vi "Read U64 Direct.vi"(8 "error in (no error)":errorcluster, 9 "Timeout (ms)":i32, 11 "CIFTag in":refnum<class "CIF_CIPC_Chn_U64.lvclass">) -> (0 "error out":errorcluster, 1 "timed out?":bool, 2 "Data":u64, 3 "CIFTag out":refnum<class "CIF_CIPC_Chn_U64.lvclass">)   [LabVIEW 2021, in "CIF_CIPC_Chn_U64.lvclass"]
uses:
  CIF_CIPC_Chn_U64.lvclass
  D:/dev/Packages/CIF_Channels_Core/src/CIFChannels/CIFChannels.lvclass
  D:/dev/Packages/CIF_Channels_Core/src/CIPC_Channels/CIF_CIPC_Chan/CIF_CIPC_Chn.lvclass
  CIFChannels/CIFChannels.lvclass/CIFChannels.ctl
  CIFChannels/Typedef/Channel State.ctl
  CIFChannels/Typedef/Direction.ctl
  CIF_CIPC_Chn_U64.lvclass/CIF_CIPC_Chn_U64.ctl
  CIF_CIPC_Chan/CIF_CIPC_Chn.lvclass/CIF_CIPC_Chn.ctl
  <vilib>/CIF Foundation/CIF CIPC/TypeDefs/Data Element Details.ctl
  ed3b2614-2534-48bf-9d55-8103b1731be4.vi
  9835d51f-0a03-4fca-8b65-57ff329e3dc0.vi
  09931085-5d07-4563-aebb-184aa810b238.vi
  a8b9b8b0-6f0e-468c-aa0e-dfff2efe2781.vi
  CIF_CIPC_Chan/Accessors/Read Buffer Configuration.vi
  CIF_CIPC_Chan/Accessors/Read Data Type.vi
  CIFChannels/Accessors/Read Channel State.vi
  CIFChannels/Accessors/Read Direction.vi
  CIFChannels/Accessors/Read Tag Forced.vi
  CIFChannels/Accessors/Write Channel State.vi
  CIFChannels/Accessors/Read Tag Disconnect Behavior.vi
  <vilib>/CIF Foundation/CIF CIPC/SubVIs/Wait For N Elements Available.vi
  <vilib>/CIF Foundation/CIF CIPC/SubVIs/Get Element Read Position.vi
  <vilib>/CIF Foundation/CIF CIPC/SubVIs/Check Error.vi
  <vilib>/CIF Foundation/CIF CIPC/SubVIs/Get dll Path.vi
  <vilib>/CIF Foundation/CIF CIPC/SubVIs/Set Element Read Position.vi
  CIF_CIPC_Chan/CIF_CIPC_Chn.lvclass
  <vilib>/Utility/error.llb/Trim Whitespace.vi
  <vilib>/Utility/error.llb/Error Cluster From Error Code.vi
  CIFChannels/CIFChannels.lvclass
  <vilib>/CIF Foundation/CIF CIPC/CIF_NI_CIPC.lvlib
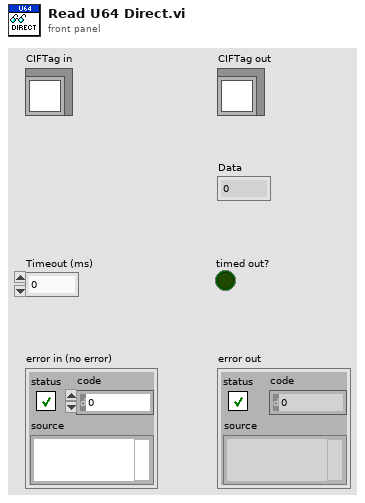
[diagram p1: front panel]
types:
  T1 = typedef "CIFChannels.lvclass/Channel State.ctl" = enum16{"Creating", "Disconnected", "Connecting", "Connected", "Destroyed"}
  T2 = typedef "CIFChannels.lvclass/Direction.ctl" = enum16{"Publisher", "Subscriber"}
  T3 = typedef "CIF_NI_CIPC.lvlib/Data Element Details.ctl" = cluster{"Bytes to Read":u32, "Element Offset":u32}
  T4 = typedef "CIF_CIPC_Chn.lvclass/Buffer Configuration Data.ctl" = cluster{"Total Size":u32, "Read Size":u32, "Read Offset":u32, "CIPC BP References":T5, "Override CIPC Name":string, "Encoder Data":string}
  T5 = typedef "CIF_NI_CIPC.lvlib/Backpressure References.ctl" = cluster{"CIPC Reference":u64, "CIPC BP Reference":u64}
  T6 = typedef "NI_Data Type.lvlib/Data Type.ctl" = enum8{"Invalid Type", "Void", "I8", "I16", "I32", "I64", "U8", "U16", "U32", "U64", "Single Float", "Double Float", "Extended Float", "Single Complex", "Double Complex", "Extended Complex", "Enum U8", "Enum U16", "Enum U32", "Enum U64", "Single Float With Unit", "Double Float With Unit", "Extended Float With Unit", "Single Complex with Unit", "Double Complex with Unit", "Extended Complex with Unit", "Boolean", "String", "Path", "Picture", "Tag", "Array", "Cluster", "Variant", "LV Variant", "Waveform", "Timestamp", "Digital Waveform", "Digital Data", "ExpressData", "Refnum", "External Data", "VI", "Poly VI", "LabVIEW Class Instance", "Fixed Point", "Set Collection", "Map Collection"}
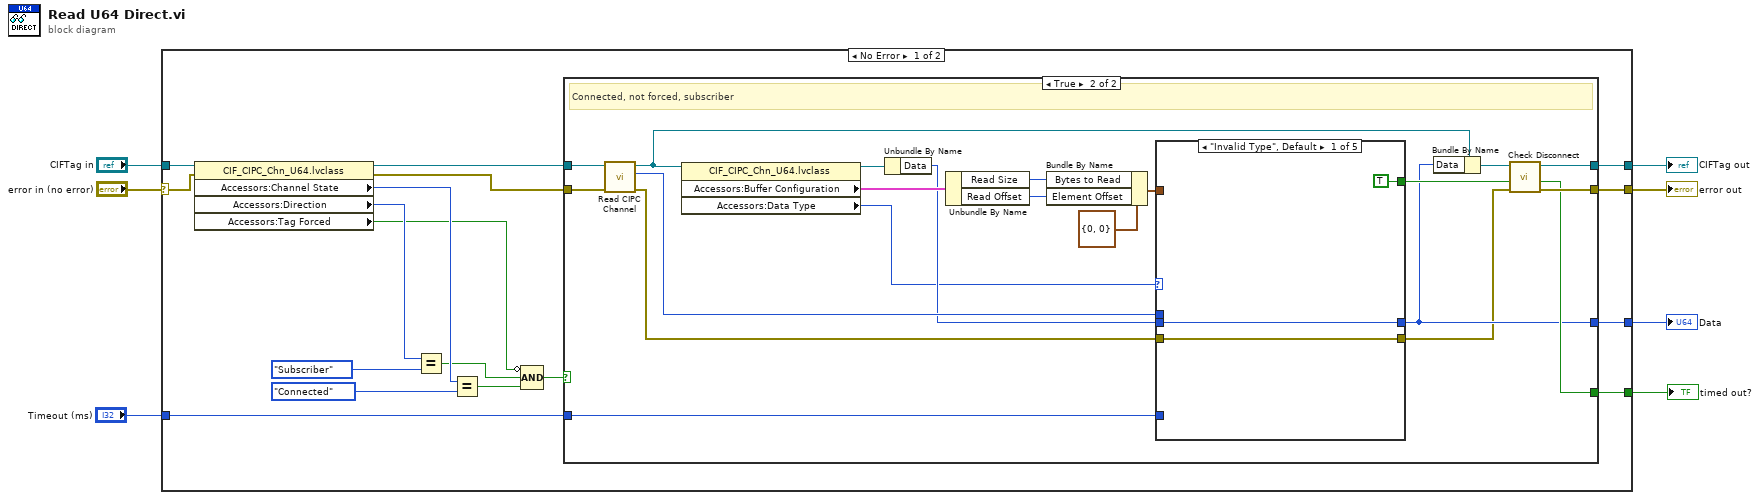
[diagram p0: block diagram]
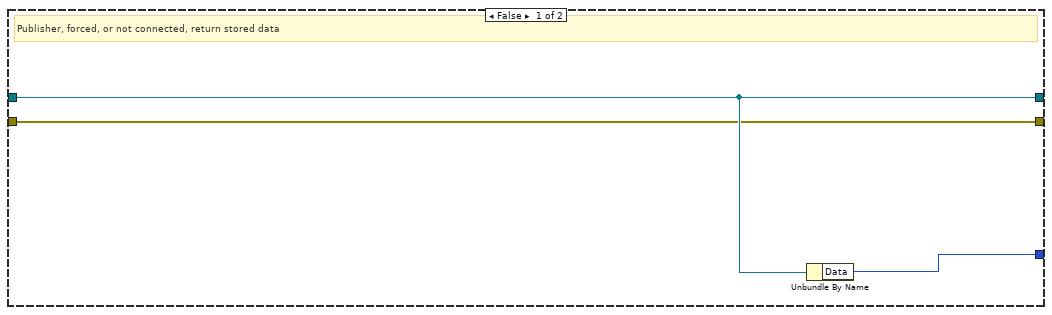
[diagram p2: hidden frame]
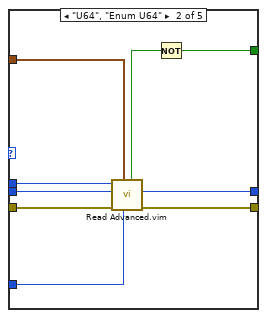
[diagram p3: hidden frame]
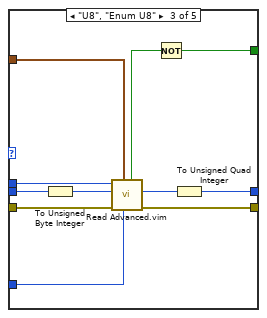
[diagram p4: hidden frame]
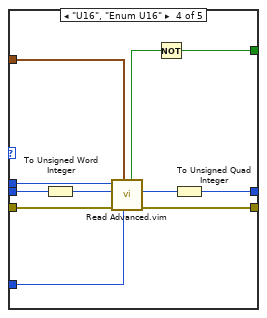
[diagram p5: hidden frame]
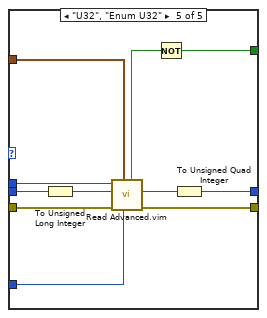
[diagram p6: hidden frame]
diagram:
  n1 = case shown="No Error" "error in (no error)" {
    selector: "error in (no error)" -> [w21 w95]
    tunnel: [w10 w95] -> w6
    tunnel: [w11 w94] -> w4
    tunnel: "CIFTag in" -> [w22 w94]
    tunnel: [w24 _] -> w3
    tunnel: [w23 _] -> w2
    tunnel: "Timeout (ms)" -> [w9 _]
    frame No Error {
      n2 = property class="CIF_CIPC_Chn_U64.lvclass"(reference=w22, error in=w21) -> (reference out=w20:refnum<class "CIF_CIPC_Chn_U64.lvclass">, error out=w19:errorcluster, "Accessors:Channel State"=w16:T1, "Accessors:Direction"=w18:T2, "Accessors:Tag Forced"=w8:bool)
      n3 = Equal?(x=w18, y=Direction."Subscriber") -> (x = y?=w12:bool)
      n4 = Equal?(x=w16, y=Channel_State."Connected") -> (x = y?=w14:bool)
      n5 = Compound Arithmetic op=AND(invert w8, w12, w14) -> (w13:bool)
      n6 = case shown="True" w13 {
        tunnel: [_ w42] -> w24
        tunnel: [w27 w31] -> w23
        tunnel: w19 -> [w25 w47]
        tunnel: w20 -> [w26 w48]
        tunnel: [w26 w45] -> w11
        tunnel: [w25 w46] -> w10
        tunnel: w9 -> [_ w32]
        frame False {
          # "Publisher, forced, or not connected, return stored data"
          n7 = Unbundle By Name(w26) -> ("Data"=w27:u64)
        }
        frame True {
          # "Connected, not forced, subscriber"
          n8 = call "Read CIPC Channel.vi"("error in (no error)"=w47, "CIFTag in"=w48) -> ("error out"=w33:errorcluster, "CIPC Channel"=w34:u64, "CIFTag out"=w41:refnum<class "CIF_CIPC_Chn_U64.lvclass">)  [unwired: 7 in]
          n9 = property class="CIF_CIPC_Chn_U64.lvclass"(reference=w41) -> (reference out=w40:refnum<class "CIF_CIPC_Chn_U64.lvclass">, "Accessors:Buffer Configuration"=w36:T4, "Accessors:Data Type"=w28:T6)  [unwired: 1 in, 1 out]
          n10 = Unbundle By Name(w40) -> ("Data"=w30:u64)
          n11 = Unbundle By Name(w36) -> ("Read Size"=w38:u32, "Read Offset"=w37:u32)
          n12 = Bundle By Name(cluster=T3 {"Bytes to Read"=0, "Element Offset"=0} ("Data Element"), "Bytes to Read"=w38, "Element Offset"=w37) -> (w35:T3)
          n13 = case shown="\"Invalid Type\", Default" w28 {
            tunnel: [TRUE w60 w71 w82 w93] -> w43
            tunnel: w35 -> [_ w59 w70 w81 w92]
            tunnel: w34 -> [_ w58 w69 w80 w91]
            tunnel: w33 -> [w50 w57 w68 w79 w90]
            tunnel: w32 -> [_ w56 w67 w78 w89]
            tunnel: [w51 w54 w61 w72 w83] -> w31
            tunnel: w30 -> [w51 w53 w64 w75 w86]
            tunnel: [w50 w52 w63 w74 w85] -> w29
            frame "Invalid Type", Default {
            }
            frame "U64", "Enum U64" {
              n14 = call "Read Advanced.vim"("Timeout (ns)"=w56, "Data Element"=w59, "error in (no error)"=w57, "Data in"=w53, "CIPC Reference in"=w58) -> ("error out"=w52:errorcluster, "Data out"=w54:u64, "Success"=w55:bool)  [unwired: 2 in, 2 out]
              n15 = Not(x=w55) -> (.not. x?=w60:bool)
            }
            frame "U8", "Enum U8" {
              n16 = To Unsigned Byte Integer(number=w64) -> (unsigned 8bit integer=w62:u8)
              n17 = call "Read Advanced.vim"("Timeout (ns)"=w67, "Data Element"=w70, "error in (no error)"=w68, "Data in"=w62, "CIPC Reference in"=w69) -> ("error out"=w63:errorcluster, "Data out"=w65:u8, "Success"=w66:bool)  [unwired: 2 in, 2 out]
              n18 = Not(x=w66) -> (.not. x?=w71:bool)
              n19 = To Unsigned Quad Integer(1:w65) -> (0:w61:u64)
            }
            frame "U16", "Enum U16" {
              n20 = To Unsigned Word Integer(number=w75) -> (unsigned 16bit integer=w73:u16)
              n21 = call "Read Advanced.vim"("Timeout (ns)"=w78, "Data Element"=w81, "error in (no error)"=w79, "Data in"=w73, "CIPC Reference in"=w80) -> ("error out"=w74:errorcluster, "Data out"=w76:u16, "Success"=w77:bool)  [unwired: 2 in, 2 out]
              n22 = Not(x=w77) -> (.not. x?=w82:bool)
              n23 = To Unsigned Quad Integer(1:w76) -> (0:w72:u64)
            }
            frame "U32", "Enum U32" {
              n24 = To Unsigned Long Integer(number=w86) -> (unsigned 32bit integer=w84:u32)
              n25 = call "Read Advanced.vim"("Timeout (ns)"=w89, "Data Element"=w92, "error in (no error)"=w90, "Data in"=w84, "CIPC Reference in"=w91) -> ("error out"=w85:errorcluster, "Data out"=w87:u32, "Success"=w88:bool)  [unwired: 2 in, 2 out]
              n26 = Not(x=w88) -> (.not. x?=w93:bool)
              n27 = To Unsigned Quad Integer(1:w87) -> (0:w83:u64)
            }
          }
          n28 = Bundle By Name(cluster=w41, "Data"=w31) -> (w44:refnum<class "CIF_CIPC_Chn_U64.lvclass">)
          n29 = call "Check Disconnect.vi"("error in (no error)"=w29, "timeout in"=w43, "CIFTag in"=w44) -> ("error out"=w46:errorcluster, "timeout out"=w42:bool, "CIFTag out"=w45:refnum<class "CIF_CIPC_Chn_U64.lvclass">)  [unwired: 5 in, 1 out]
        }
      }
    }
    frame Error {
    }
  }
  "error out" <- w6
  "CIFTag out" <- w4
  "timed out?" <- w3
  "Data" <- w2
